vi "Read Drive Motor Setpoints.vi"(1 "Input Array":dbl[](array[numeric])) -> (0 "Appended Array":dbl[](array[numeric]))   [LabVIEW 2014]
uses:
  Begin/Global Variables.vi
panel:
  out "Drive BR Setspeed":dbl
  out "Drive BL Setspeed":dbl
  out "Drive FR Setspeed":dbl
  out "Drive FL Setspeed":dbl
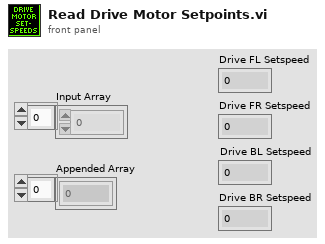
[diagram p1: front panel]
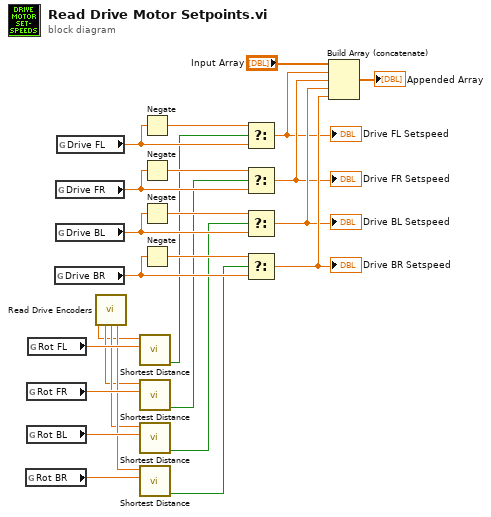
[diagram p0: block diagram]
diagram:
  n1 = global read "Global Variables.vi" "Rot BR"() -> (w23:dbl)
  n2 = global read "Global Variables.vi" "Rot FR"() -> (w25:dbl)
  n3 = global read "Global Variables.vi" "Rot BL"() -> (w24:dbl)
  n4 = global read "Global Variables.vi" "Rot FL"() -> (w26:dbl)
  n5 = global read "Global Variables.vi" "Drive BR"() -> (w18:dbl)
  n6 = global read "Global Variables.vi" "Drive FR"() -> (w16:dbl)
  n7 = global read "Global Variables.vi" "Drive BL"() -> (w17:dbl)
  n8 = global read "Global Variables.vi" "Drive FL"() -> (w15:dbl)
  n9 = call "Read Drive Encoders.vi"() -> ("Drive Encoder BR"=w4:dbl, "Drive Encoder BL"=w3:dbl, "Drive Encoder FR"=w2:dbl, "Drive Encoder FL"=w1:dbl)  [unwired: 11 in, 1 out]
  n10 = call "Shortest Distance.vi"("target"=w26, "current"=w1) -> ("flipping?"=w14:bool)  [unwired: 8 in, 1 out]
  n11 = call "Shortest Distance.vi"("target"=w25, "current"=w2) -> ("flipping?"=w13:bool)  [unwired: 8 in, 1 out]
  n12 = call "Shortest Distance.vi"("target"=w24, "current"=w3) -> ("flipping?"=w12:bool)  [unwired: 8 in, 1 out]
  n13 = call "Shortest Distance.vi"("target"=w23, "current"=w4) -> ("flipping?"=w11:bool)  [unwired: 8 in, 1 out]
  n14 = Negate(x=w15) -> (-x=w22:dbl)
  n15 = Negate(x=w16) -> (-x=w19:dbl)
  n16 = Negate(x=w17) -> (-x=w20:dbl)
  n17 = Negate(x=w18) -> (-x=w21:dbl)
  n18 = Select(t=w22, s=w14, f=w15) -> (s? t:f=w5:dbl)
  "Drive FL Setspeed" <- w5
  n19 = Select(t=w19, s=w13, f=w16) -> (s? t:f=w6:dbl)
  "Drive FR Setspeed" <- w6
  n20 = Select(t=w20, s=w12, f=w17) -> (s? t:f=w7:dbl)
  "Drive BL Setspeed" <- w7
  n21 = Select(t=w21, s=w11, f=w18) -> (s? t:f=w8:dbl)
  "Drive BR Setspeed" <- w8
  n22 = Build Array (concatenate)("Input Array", w5, w6, w7, w8) -> (→"Appended Array":dbl[])
